vi "UnflattenFromString.vi"(8 "error in (no error)":errorcluster, 10 "String in":string, 11 "dvotAFTKinetics in":refnum<class "dvotAFTKinetics.lvclass">) -> (0 "error out":errorcluster, 3 "dvotAFTKinetics out":refnum<class "dvotAFTKinetics.lvclass">)   [LabVIEW 2012, in "dvotAFTKinetics.lvclass"]
uses:
  dvotAFTKinetics.lvclass
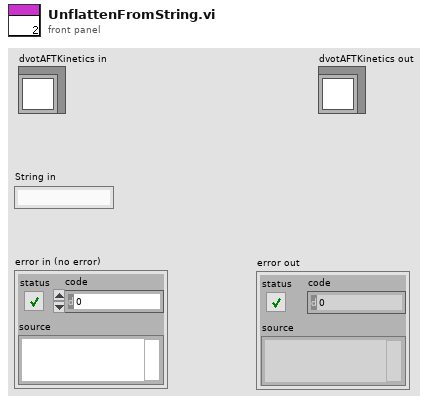
[diagram p1: front panel]
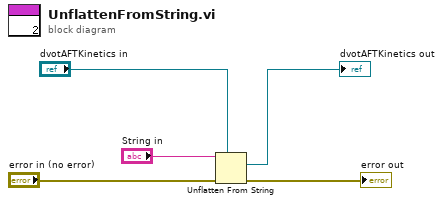
[diagram p0: block diagram]
diagram:
  n1 = Unflatten From String(type="dvotAFTKinetics in", binary string="String in", error in (no error)="error in (no error)") -> (value=→"dvotAFTKinetics out":refnum<class "dvotAFTKinetics.lvclass">, error out=→"error out":errorcluster)  [unwired: 2 in, 1 out]
